vi "PrimaryInterfaceGetVariableByName.vi"(8 "name":string, 9 "PrimaryInterface":refnum<k24>, 11 "error in":errorcluster) -> (0 "Variable":refnum<k24>, 1 "Value":T1, 2 "Exists":bool, 3 "error out":errorcluster)   [LabVIEW 2022 SP3, in "UnderAutomation.UniversalRobots.lvlib"]
uses:
  UnderAutomation.UniversalRobots.lvlib
  C:/Users/fg/Documents/UniversalRobots.vi/LabVIEW_2023/UnderAutomation.UniversalRobots/lib/UnderAutomation.UniversalRobots.dll
  LabVIEW_2023/UnderAutomation.UniversalRobots/lib/UnderAutomation.UniversalRobots.dll
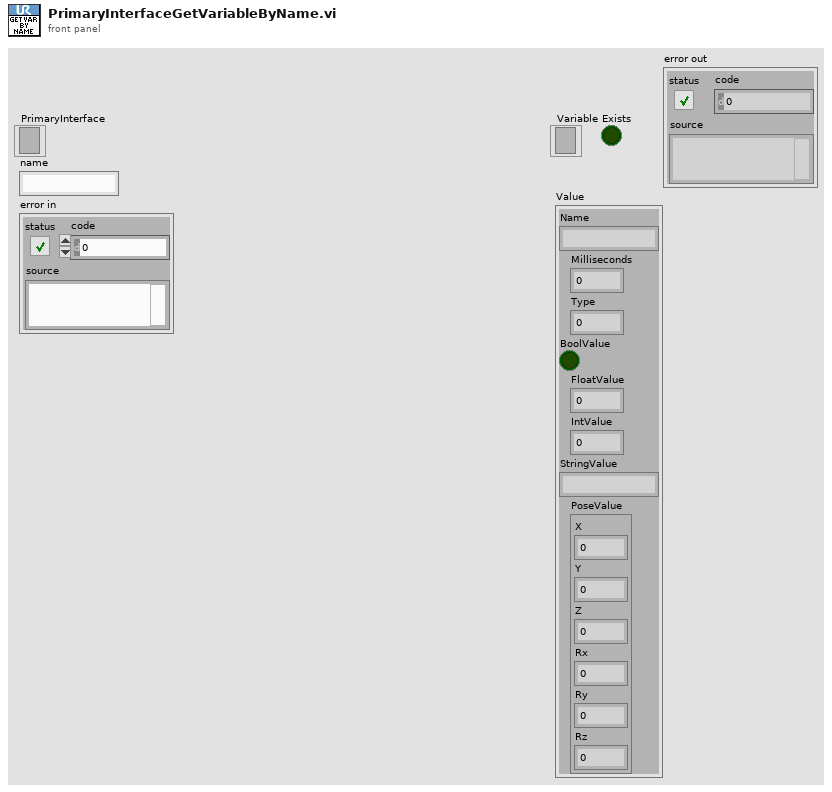
[diagram p1: front panel]
types:
  T1 = cluster{"Name":string, "Milliseconds":i32, "Type":i32, "BoolValue":bool, "FloatValue":sgl, "IntValue":i32, "StringValue":string, "PoseValue":cluster{"X":dbl, "Y":dbl, "Z":dbl, "Rx":dbl, "Ry":dbl, "Rz":dbl}}
  T2 = cluster{"Name":string, "Milliseconds":i32, "Type":i32, "ToBool":bool, "ToFloat":sgl, "ToInt":i32, "ToString":string, cluster{"X":dbl, "Y":dbl, "Z":dbl, "Rx":dbl, "Ry":dbl, "Rz":dbl}}
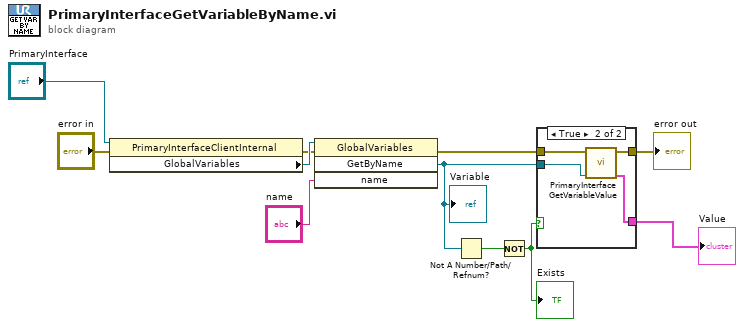
[diagram p0: block diagram]
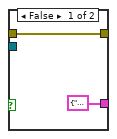
[diagram p2: hidden frame]
diagram:
  n1 = property class="PrimaryInterfaceClientInternal"(reference="PrimaryInterface", error in="error in") -> (error out=w6:errorcluster, "GlobalVariables"=w10:refnum<k24>)  [unwired: 1 out]
  n2 = invoke class="GlobalVariables" method="GetByName"(reference=w10, error in=w6, "name"="name") -> (error out=w4:errorcluster, "GetByName"=w3:refnum<k24>)  [unwired: 1 in, 2 out]
  "Variable" <- w3
  n3 = Not A Number/Path/Refnum?(number/path/refnum=w3) -> (NaN/Path/Refnum?=w8:bool)
  n4 = Not(x=w8) -> (.not. x?=w5:bool)
  "Exists" <- w5
  n5 = case shown="True" w5 {
    tunnel: w4 -> [w12 w17]
    tunnel: w3 -> [_ w16]
    tunnel: [T2 {"Name"="", "Milliseconds"=0, "Type"=0, "ToBool"=FALSE, "ToFloat"=0.0, "ToInt"=0, "ToString"="", {"X"=0.0, "Y"=0.0, "Z"=0.0, "Rx"=0.0, "Ry"=0.0, "Rz"=0.0}} ("Value") w15] -> w2
    tunnel: [w12 w14] -> w1
    frame False {
    }
    frame True {
      n6 = call "PrimaryInterfaceGetVariableValue.vi"("Variable"=w16, "error in"=w17) -> ("Value"=w15:T1, "error out"=w14:errorcluster)  [unwired: 8 in]
    }
  }
  "error out" <- w1
  "Value" <- w2
